vi "motor fpga PID test 002.vi"() -> ()   [LabVIEW 2019]
uses:
  motor single class/Variable PID(Kp).ctl
  motor single class/Variable PID(Kp) mode enum.ctl
  motor single class/Motor single.lvclass
  motor enum(FPGA).ctl
  <vilib>/Platform/TimedLoop/XDataNode/timing_clust.ctl
  <vilib>/Platform/TimedLoop/XDataNode/nitl_modes.ctl
  <vilib>/Platform/TimedLoop/XDataNode/wakeup.ctl
  <vilib>/platform/TimedLoop/XDataNode/XDataNode.xnode
  <vilib>/Platform/TimedLoop/XDataNode/XDNodeRunTimeDep.lvlib
panel:
  in  "stop":bool
  in  "Array":dbl[](array[slide])=[0.0, 0.0, -4.0697674418604635] scale=-125.0..125.0
  out "error out":errorcluster
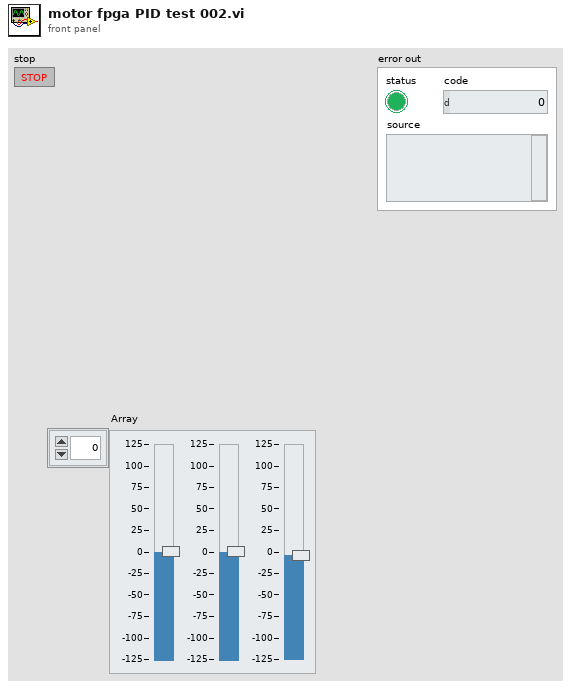
[diagram p1: front panel]
types:
  T1 = typedef "Motor single.lvclass/motor enum(FPGA).ctl" = enum16{"M1", "M2", "M3", "M4"}
  T2 = typedef "Motor single.lvclass/Variable PID(Kp).ctl" = cluster{"Enable variable PID(Kp)":bool, "Variable PID(Kp)range":dbl, "Variable MODE":T3}
  T3 = typedef "Motor single.lvclass/Variable PID(Kp) mode enum.ctl" = enum16{"Log", "Sin&Cos", "Linear", "reverse Log", "const"}
  T4 = typedef "XDNodeRunTimeDep.lvlib/timing_clust.ctl" = cluster{"Expected End [f-1]":u64, "Actual End [f-1]":u64, "Finished Late? [f-1]":bool, "Expected End [i-1]":u64, "Actual End [i-1]":u64, "Finished Late? [i-1]":bool, "Expected Start [i]":u64, "Actual Start [i]":u64, "Expected Start [f]":u64, "Actual Start [f]":u64, "Source Name":string, "Structure Name":string, "Period":i64, "Deadline":i64, "Offset":i64, "Start":i64, "Priority":i32, "Timeout":i32, "Mode":T5, "Wakeup Reason":T6, "Error":errorcluster, "Source Type":string, "Secondary Source Type":string, "Global End Time":u64, "Global Start Time":u64, "Frame Duration":u64, "Iteration Duration":u64, "Assigned CPU":i32, "I/O Scan Engine Mode":u32}
  T5 = typedef "XDNodeRunTimeDep.lvlib/nitl_modes.ctl" = enum32{"No Change", "Process missed periods, maintain original phase", "Discard missed periods, maintain original phase", "Process missed periods, ignore original phase", "Discard missed periods, ignore original phase"}
  T6 = typedef "XDNodeRunTimeDep.lvlib/wakeup.ctl" = enum32{"Normal", "Aborted", "Asynchronous wakeup", "Timing source error", "Timed loop error", "Timeout"}
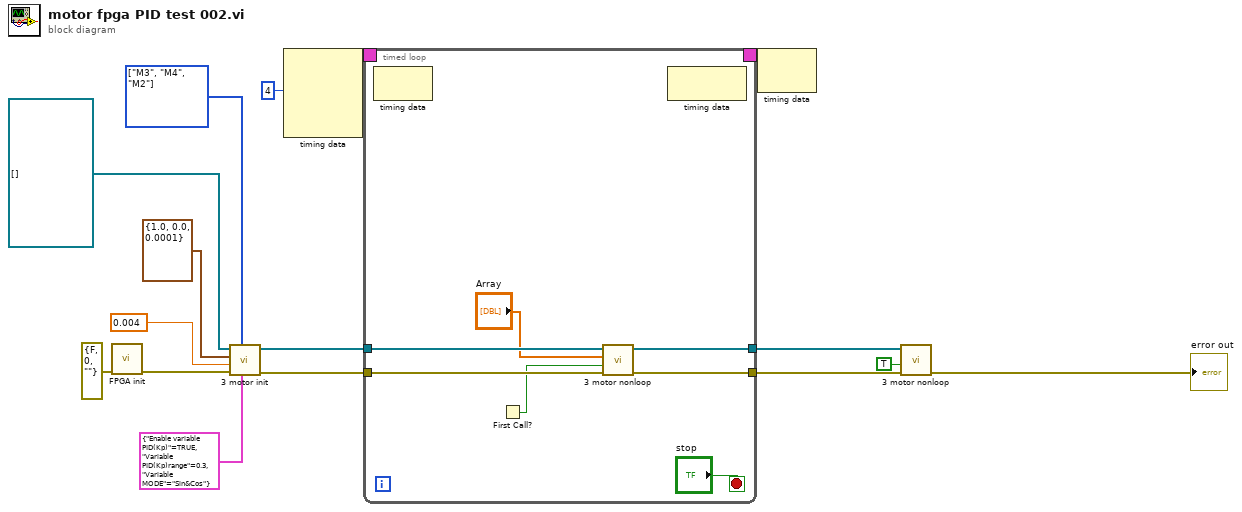
[diagram p0: block diagram]
diagram:
  w3 = T1[] [enum."M3", enum."M4", enum."M2"] items=["M1", "M2", "M3", "M4"] ("Array 2")
  n1 = call "FPGA init.vi"("error in"=errorcluster {"status"=FALSE, "code"=0, "source"=""}) -> ("error out"=w8:errorcluster)  [unwired: 9 in, 1 out]
  n2 = call "3 motor init.vi"("Variable PID(Kp)"=T2 {"Enable variable PID(Kp)"=TRUE, "Variable PID(Kp)range"=0.3, "Variable MODE"=enum."Sin&Cos"}, "Array 2"=w3, "Error In"=w8, "dt(s)"=0.004, "PID"=cluster{"Kp":dbl, "Ki":dbl, "Kd":dbl} {"Kp"=1.0, "Ki"=0.0, "Kd"=0.0001}, "Array"=refnum<class "Motor single.lvclass">[] []) -> ("error out"=w13:errorcluster, "Object array"=w14:refnum<class "Motor single.lvclass">[])  [unwired: 4 in]
  n3 = node-c288(i64 4 ("Period")) -> (w16:T4)  [unwired: 3 in]
  n4 = timed-loop {
    timing: w16 -> [_]
    timing-out: [_] -> w15
    tunnel: w14 -> [w23]
    tunnel: w13 -> [w22]
    tunnel: [w20] -> w12
    tunnel: [w19] -> w11
    stop <- "stop" stop-if-true
    n5 = node-c288() -> ()  [unwired: 1 in, 1 out]
    n6 = First Call?() -> (First Call?: T/F=w21:bool)
    n7 = call "3 motor nonloop.vi"("Error In"=w22, "Reset"=w21, "speed"="Array", "Array"=w23) -> ("error out"=w20:errorcluster, "appended array"=w19:refnum<class "Motor single.lvclass">[])  [unwired: 3 in, 3 out]
    n8 = node-c288() -> ()  [unwired: 1 in, 1 out]
  }
  n9 = node-c288(w15) -> ()  [unwired: 1 out]
  n10 = call "3 motor nonloop.vi"("Error In"=w12, "Reset"=TRUE, "Array"=w11) -> ("error out"=→"error out":errorcluster)  [unwired: 4 in, 4 out]
